vi "InitDone.vi"(8 "error in (no error)":errorcluster, 9 "InstrumentData":T1, 10 "Boolean":bool, 11 "SpectroscopyUI in":refnum<class "SpectroscopyUI.lvclass">) -> (0 "error out":errorcluster, 3 "SpectroscopyUI out":refnum<class "SpectroscopyUI.lvclass">)   [LabVIEW 2023, in "SpectroscopyUI.lvlib" / "SpectroscopyUI.lvclass"]
uses:
  SpectroscopyUI.lvclass
  SpectroscopyUI.lvclass/SpectroscopyUI.ctl
  InterferometryUI/InterferometryUI/instrumentType.ctl
  ConcreteClasses/ConcreteInstrumentClasses/CameraClasses/Hama_LV/HamaCam/HamaCam/InstrumentData.ctl
panel:
  in  "instr error":errorcluster
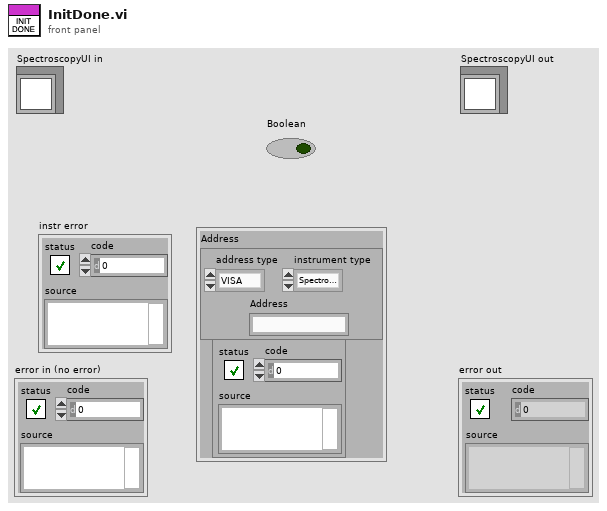
[diagram p1: front panel]
types:
  T1 = typedef "InstrumentData.ctl" = cluster{"Instr Error":errorcluster, "Address":cluster{"address type":enum16{"VISA", "Index"}, "Address":string, "instrument type":T2}}
  T2 = typedef "instrumentType.ctl" = enum16{"Spectrometer", "Camera", "Stepper"}
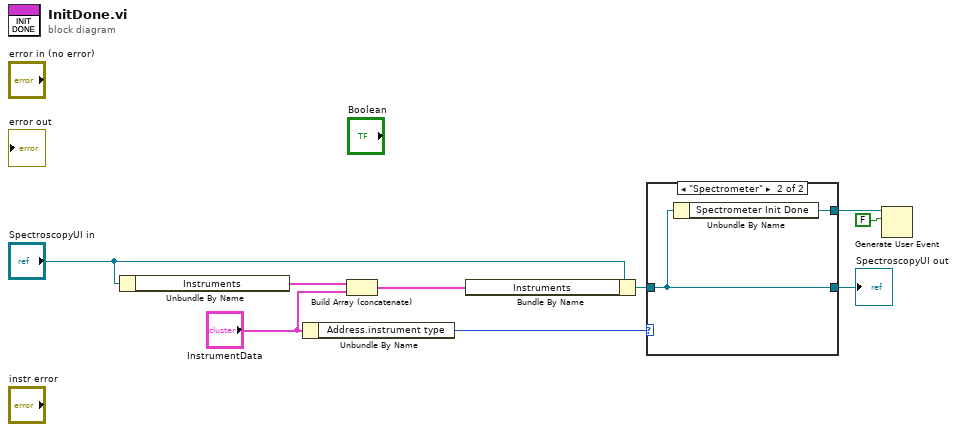
[diagram p0: block diagram]
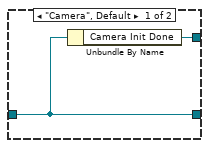
[diagram p2: hidden frame]
diagram:
  n1 = Unbundle By Name("SpectroscopyUI in") -> ("Instruments"=w5:T1[])
  n2 = Unbundle By Name("InstrumentData") -> ("Address.instrument type"=w9:T2)
  n3 = Build Array (concatenate)(w5, "InstrumentData") -> (w4:T1[])
  n4 = Bundle By Name(cluster="SpectroscopyUI in", "Instruments"=w4) -> (w1:refnum<class "SpectroscopyUI.lvclass">)
  n5 = case shown="\"Spectrometer\"" w9 {
    tunnel: [w11 w13] -> w7
    tunnel: [w10 w12] -> w8
    tunnel: w1 -> [w10 w12]
    frame "Camera", Default {
      n6 = Unbundle By Name(w10) -> ("Camera Init Done"=w11:refnum<user-event>)
    }
    frame "Spectrometer" {
      n7 = Unbundle By Name(w12) -> ("Spectrometer Init Done"=w13:refnum<user-event>)
    }
  }
  "SpectroscopyUI out" <- w8
  n8 = Generate User Event(user event=w7, event data cluster=FALSE ("event data")) -> ()  [unwired: 2 in, 2 out]
